vi "Query.vi"(8 "error in (no error)":errorcluster, 10 "Command":string=":measure:", 11 "Reference in":T1={"Device"="GPIB0::4::INSTR", "Function"="", "delay"=20}) -> (0 "error out":errorcluster, 2 "Answer":string, 3 "Reference out":T1={"Device"="GPIB0::4::INSTR", "Function"="", "delay"=20}, 4 "question out":string)   [LabVIEW 2021, in "Rigol DM3052.lvlib"]
uses:
  Rigol DM3052.lvlib
  Reference.ctl
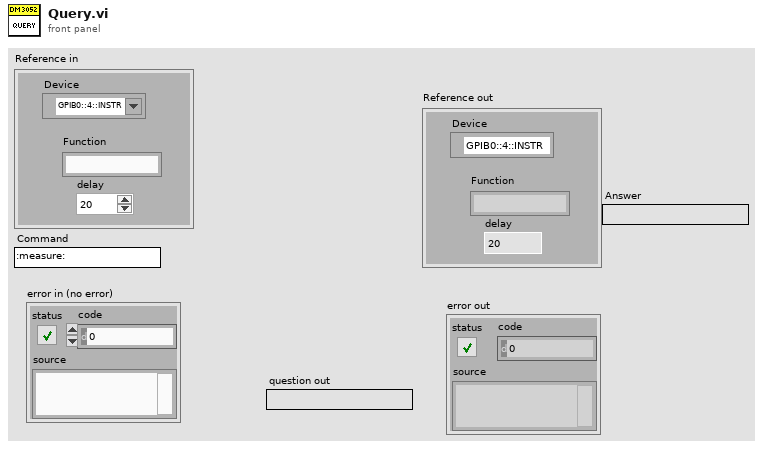
[diagram p1: front panel]
types:
  T1 = typedef "Rigol DM3052.lvlib/Reference.ctl" = cluster{"Device":refnum<visa-resource-name>, "Function":string, "delay":u32}
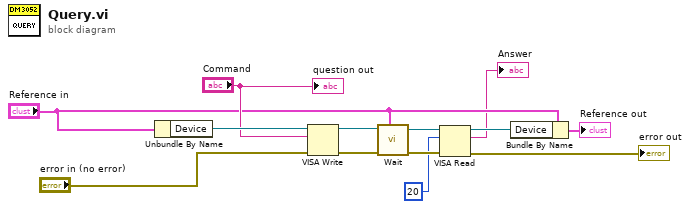
[diagram p0: block diagram]
diagram:
  n1 = Unbundle By Name("Reference in") -> ("Device"=w13:refnum<visa-resource-name>)
  n2 = VISA Write(VISA resource name=w13, write buffer="Command", error in (no error)="error in (no error)") -> (VISA resource name out=w10:refnum<visa-resource-name>, error out=w9:errorcluster)  [unwired: 1 out]
  n3 = call "Wait.vi"("Reference in"="Reference in", "error in (no error)"=w9, "Device in"=w10) -> ("error out"=w7:errorcluster, "Device out"=w8:refnum<visa-resource-name>)  [unwired: 7 in]
  n4 = VISA Read(VISA resource name=w8, byte count=u32 20, error in (no error)=w7) -> (VISA resource name out=w5:refnum<visa-resource-name>, read buffer=→"Answer":string, error out=→"error out":errorcluster)  [unwired: 1 out]
  n5 = Bundle By Name(cluster="Reference in", "Device"=w5) -> (→"Reference out":T1)
  "question out" <- "Command"
